vi "ToEnum.vi"(8 "error in":errorcluster, 11 "Ring in":refnum<class "Generic.lvclass">) -> (0 "error out":errorcluster, 3 "Enum out":refnum<class "Enum.lvclass">)   [LabVIEW 2014, in "Raspberry Pi Compatible Compiler for LabVIEW.lvlib" / "Enum.lvclass"]
uses:
  Enum.lvclass
  Generic/Generic.lvclass
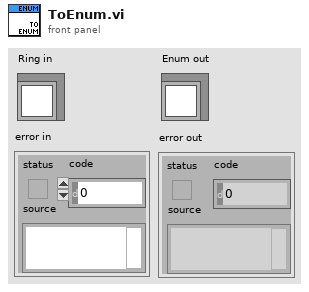
[diagram p1: front panel]
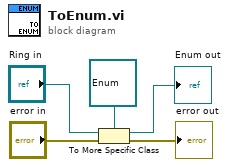
[diagram p0: block diagram]
diagram:
  n1 = To More Specific Class(target class=refnum<class "Enum.lvclass"> refnum ("Ring in"), reference="Ring in", error in="error in") -> (specific class reference=→"Enum out":refnum<class "Enum.lvclass">, error out=→"error out":errorcluster)
